vi "Get All Wires.vi"(0 "Diagram In":refnum<vi>, 1 "error in":errorcluster) -> (2 "Diagram Out":refnum<vi>, 3 "All Wires":refnum<vi>[](array[refnum]), 4 "error out":errorcluster)   [LabVIEW 2012, in "Scripting Tools.lvlib"]
doc: "Returns all GObjects from the block diagram referenced by <B>Diagram In</B>, including all those in sub-diagrams (loops and sequence structures etc)."
uses:
  Scripting Tools.lvlib
  <vilib>/Utility/traverseref.llb/TRef TravTarget.ctl
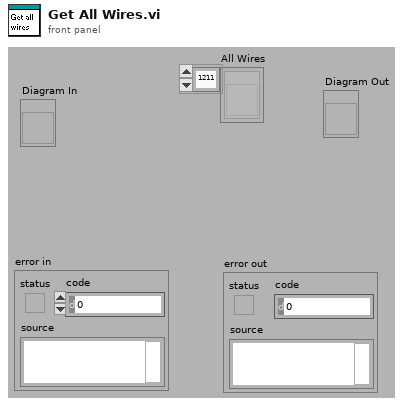
[diagram p1: front panel]
types:
  T1 = typedef "TRef TravTarget.ctl" = enum16{"FP", "BD", "Other"}
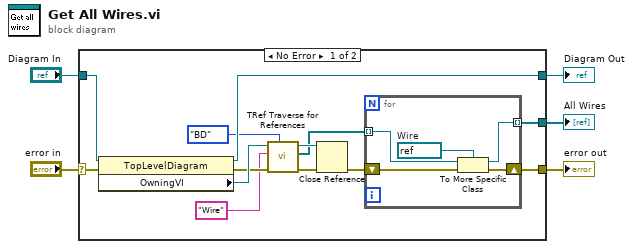
[diagram p0: block diagram]
diagram:
  n1 = case shown="No Error" "error in" {
    selector: "error in" -> [w16 w25]
    tunnel: [w7 w25] -> w5
    tunnel: "Diagram In" -> [w18 w24]
    tunnel: [w17 w24] -> w3
    tunnel: [w6 _] -> w1
    frame No Error {
      n2 = property on="Property Node" class="TopLevelDiagram"(reference=w18, error in=w16) -> (reference out=w17:refnum<vi>, error out=w14:errorcluster, "OwningVI"=w15:refnum<vi>)
      n3 = call <vilib>:"TRef Traverse for References.vi"("Traverse Target"=TRef_TravTarget."BD", "error in (no error)"=w14, "Class Name"="Wire", "VI Refnum"=w15) -> ("error out"=w13:errorcluster, "References"=w8:refnum<vi>[], "dup VI Refnum"=w12:refnum<vi>)  [unwired: 1 in, 4 out]
      n4 = Close Reference(reference=w12, error in (no error)=w13) -> (error out=w9:errorcluster)
      n5 = for {
        shift-right: [w22] -> w7
        shift-left: w9 -> [w23]
        tunnel: w8 -> [w21] mode=indexing
        tunnel: [w19] -> w6 mode=indexing
        w20 = refnum<vi> refnum  # Wire
        n6 = To More Specific Class(target class=w20, reference=w21, error in=w23) -> (specific class reference=w19:refnum<vi>, error out=w22:errorcluster)
      }
    }
    frame Error {
    }
  }
  "error out" <- w5
  "Diagram Out" <- w3
  "All Wires" <- w1
